vi "setEventSettingsApplied.vi"(10 "EventSettingsApplied":T1, 11 "Publisher in":refnum<class "Publisher.lvclass">) -> (3 "Publisher out":refnum<class "Publisher.lvclass">)   [LabVIEW 2016, in "Publisher.lvclass"]
uses:
  Publisher.lvclass
  DataTypes/Topics/EventSettingsApplied.ctl
  DataTypes/Topics/Parts/Timestamp.ctl
  Publisher.lvclass/Publisher.ctl
  DataTypes/Topics/M1M3SupportTopics.lvlib
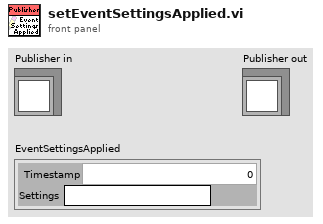
[diagram p1: front panel]
types:
  T1 = typedef "M1M3SupportTopics.lvlib/EventSettingsApplied.ctl" = cluster{"Timestamp":T2, "Settings":string}
  T2 = typedef "M1M3SupportTopics.lvlib/Timestamp.ctl" = dbl
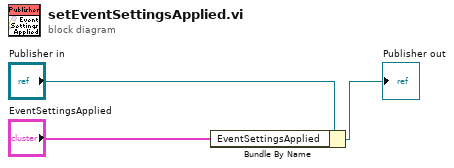
[diagram p0: block diagram]
diagram:
  n1 = Bundle By Name(cluster="Publisher in", "EventSettingsApplied"="EventSettingsApplied") -> (→"Publisher out":refnum<class "Publisher.lvclass">)
